vi "readCellValue.vi"(8 "error in (no error)":errorcluster) -> (0 "error out":errorcluster, 3 "resulting string":string)   [LabVIEW 2023]
panel:
  out "chiffre":i32
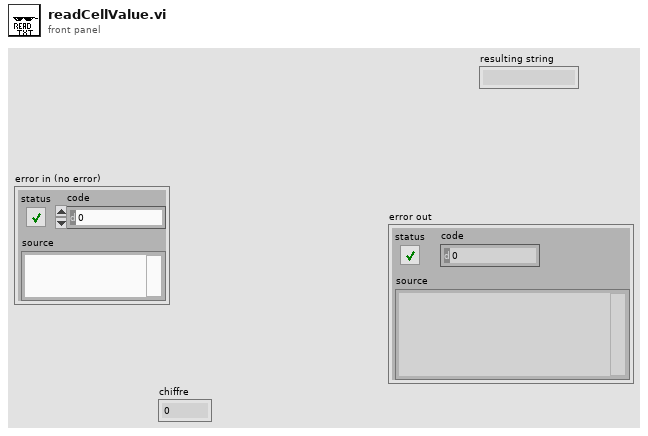
[diagram p1: front panel]
types:
  T1 = enum16{"open", "replace", "create", "open or create", "replace or create", "replace or create with confirmation"}
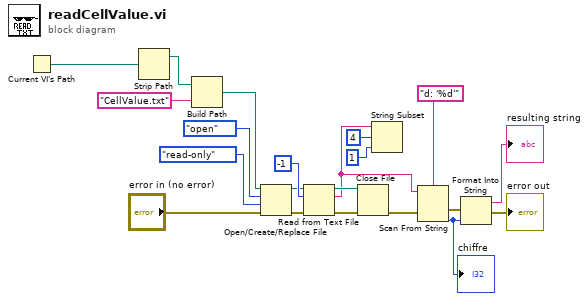
[diagram p0: block diagram]
diagram:
  n1 = Current VI's Path() -> (path=w20:path)
  n2 = Strip Path(path=w20) -> (stripped path=w21:path)  [unwired: 1 out]
  n3 = Build Path(base path=w21, name or relative path="CellValue.txt") -> (appended path=w19:path)
  n4 = Open/Create/Replace File(file path (use dialog)=w19, error in="error in (no error)", operation (0:open)=T1."open", access (0:read/write)=enum16{"read/write", "read-only", "write-only"}."read-only") -> (refnum out=w7:refnum<file>, error out=w14:errorcluster)  [unwired: 2 in, 1 out]
  n5 = Read from Text File(file (use dialog)=w7, count=-1, error in=w14) -> (refnum out=w6:refnum<file>, text=w1:string, error out=w13:errorcluster)  [unwired: 1 in, 1 out]
  n6 = Close File(refnum=w6, error in=w13) -> (error out=w5:errorcluster)  [unwired: 1 out]
  n7 = String Subset(string=w1, offset (0)=4, length (rest)=1 ("length (rest)")) -> ()  [unwired: 1 out]
  n8 = Scan From String(format string="d: '%d'", input string=w1, error in=w5) -> (error out=w4:errorcluster, output 1=w3:i32)  [unwired: 2 in, 2 out]
  "chiffre" <- w3
  n9 = Format Into String(error in=w4, w3) -> (resulting string=→"resulting string":string, error out=→"error out":errorcluster)  [unwired: 2 in]
